vi "DLTS - modify pluse (SubVI).vi"(8 "error in (no error)":errorcluster, 9 "AUX scale":dbl[unit], 10 "TUpulse on time":dbl[unit], 11 "Handle Out in":T1 {"Handle" format="0x%08x"; "Conn" format="0x%08x"}) -> (0 "error out":errorcluster, 3 "Handle Out out":T1 {"Handle" format="0x%08x"; "Conn" format="0x%08x"})   [LabVIEW 2019]
doc: "Configures DLTS biasing pulse timing"
uses:
  <instrlib>/Zurich Instruments LabOne/Zurich Instruments LabOne.lvlib
  <instrlib>/Zurich Instruments LabOne/Public/Configure/ziSetValueDoubleArray.vi
  <instrlib>/Zurich Instruments LabOne/Public/ziTypeHandle.ctl
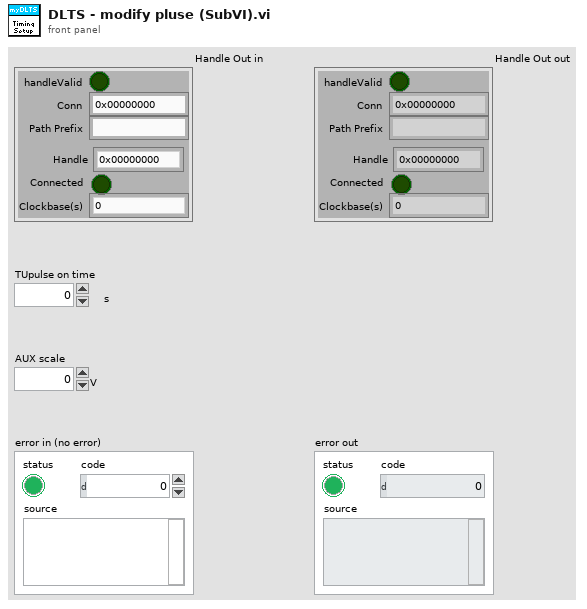
[diagram p1: front panel]
types:
  T1 = typedef "Zurich Instruments LabOne.lvlib/ziTypeHandle.ctl" = cluster{"handleValid":bool, "Conn":u64, "Path Prefix":string, "Handle":u64, "Connected":bool, "Clockbase(s)":dbl}
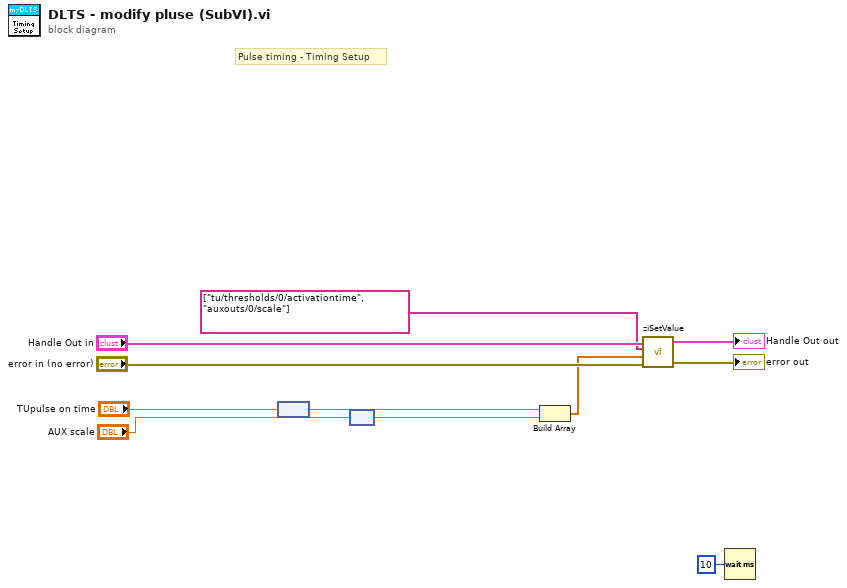
[diagram p0: block diagram]
diagram:
  # "Pulse timing - Timing Setup"
  n1 = node("TUpulse on time") -> (w2:dbl)
  n2 = node("AUX scale") -> (w1:dbl)
  n3 = Build Array(w2, w1) -> (w5:dbl[])
  n4 = call-poly <instrlib>:"ziSetValue.vi"("Error In"="error in (no error)", "Values"=w5, "Paths"=string[] ["tu/thresholds/0/activationtime", "auxouts/0/scale"], "Handle In"="Handle Out in") -> ("Error Out"=→"error out":errorcluster, "Handle Out"=→"Handle Out out":T1)  [unwired: 1 in]
  n5 = Wait (ms)(milliseconds to wait=u32 10) -> ()  [unwired: 1 out]
